vi "get_TIFF_Page.vi"(8 "error in (no error)":errorcluster, 10 "page":i32, 11 "path in":path) -> (0 "error out":errorcluster, 1 "data 32bit":u32[][](array[numeric]), 2 "data 16bit":u16[][](array[numeric]), 3 "path out":path, 4 "bits per sample":u16, 5 "data 8bit":u8[][](array[numeric]), 6 "samples per pixel":i32)   [LabVIEW 2010, in "TIFFManagement.lvlib"]
uses:
  TIFFManagement.lvlib
  VisualCPP/Release/TIFFManagement.dll
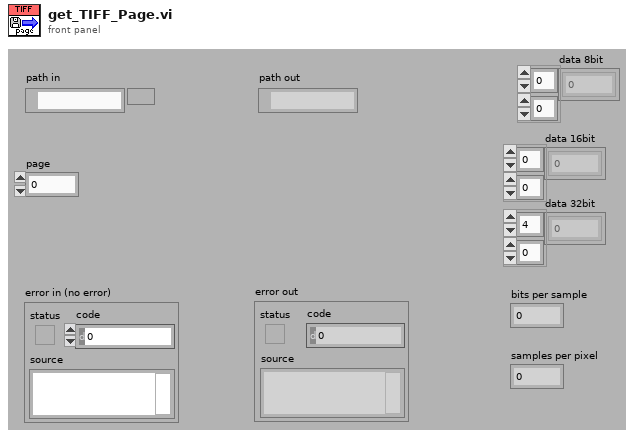
[diagram p1: front panel]
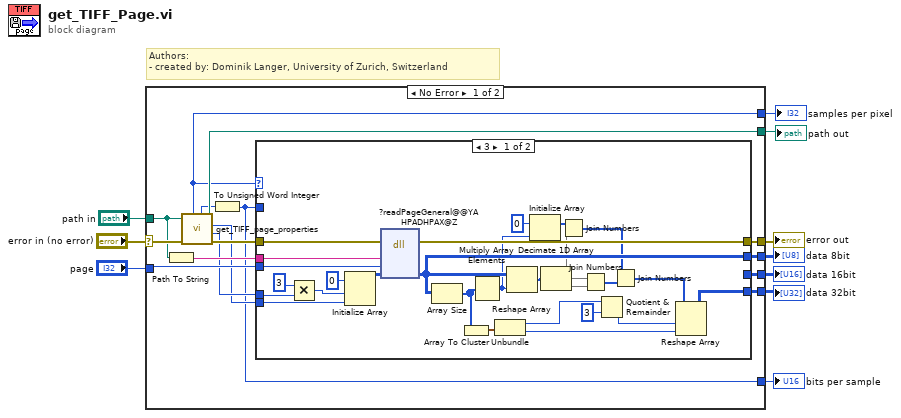
[diagram p0: block diagram]
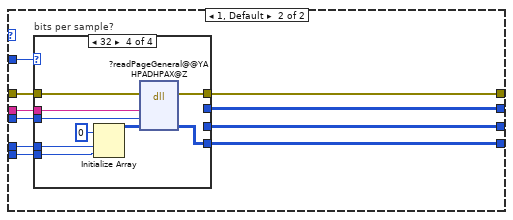
[diagram p2: hidden frame]
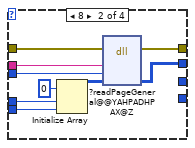
[diagram p4: hidden frame]
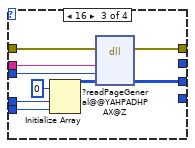
[diagram p5: hidden frame]
diagram:
  # "Authors: \n- created by: Dominik Langer, University of Zurich, Switzerland"
  n1 = case shown="No Error" "error in (no error)" {
    selector: "error in (no error)" -> [w23 w93]
    tunnel: "path in" -> [w21 w92]
    tunnel: "page" -> [w19 _]
    tunnel: [w25 w93] -> w7
    tunnel: [w20 w92] -> w6
    tunnel: [w16 _] -> w5
    tunnel: [w15 _] -> w4
    tunnel: [w14 _] -> w3
    tunnel: [w12 _] -> w2
    tunnel: [w11 _] -> w1
    frame No Error {
      n2 = Path To String(path=w21) -> (string=w24:string)
      n3 = call "get_TIFF_page_properties.vi"("error in (no error)"=w23, "path in"=w21) -> ("error out"=w22:errorcluster, "height"=w18:i32, "width"=w17:i32, "path out"=w20:path, "bits per sample"=w13:i32, "samples per pixel"=w11:i32)  [unwired: 3 in, 1 out]
      n4 = To Unsigned Word Integer(number=w13) -> (unsigned 16bit integer=w12:u16)
      n5 = case shown="3" w11 {
        tunnel: [w52 w63] -> w25
        tunnel: w24 -> [w50 w62]
        tunnel: w22 -> [w53 w61]
        tunnel: w19 -> [w49 w60]
        tunnel: w18 -> [w46 w59]
        tunnel: w17 -> [w51 w58]
        tunnel: [_ w57] -> w16
        tunnel: [w39 w56] -> w15
        tunnel: [w37 w55] -> w14
        tunnel: w12 -> [_ w54]
        frame 3 {
          n6 = Multiply(x=3 ("y"), y=w46) -> (x*y=w45:i32)
          n7 = Initialize Array(u8 0 ("element"), w45, w51) -> (w47:u8[][])
          n8 = dll-call lib="C:/helioscan/common/libraries/TIFFManagement/VisualCPP/Release/TIFFManagement.dll" fn="?readPageGeneral@@YAHPADHPAX@Z"(error in=w53, "path"=w50, "page"=w49, "data"=w47) -> (error out=w52:errorcluster, "data"=w39:u8[][])  [unwired: 5 in, 1 out]
          n9 = Array Size(array=w39) -> (size(s)=w41:i32[])
          n10 = Array To Cluster(array=w41) -> (cluster=w42:cluster{"[0]":i32, "[1]":i32})
          n11 = Multiply Array Elements(1:w41) -> (0:w29:i32)
          n12 = Unbundle(w42) -> ("[0]"=w27:i32, "[1]"=w43:i32)
          n13 = Reshape Array(w39, w29) -> (w40:u8[])
          n14 = Initialize Array(u8 0 ("element"), w29) -> (w31:u8[])
          n15 = Decimate 1D Array(w40) -> (w32:u8[], w36:u8[], w35:u8[])
          n16 = Join Numbers(hi=w31, lo=w32) -> ((hi.lo)=w30:u16[])
          n17 = Join Numbers(hi=w36, lo=w35) -> ((hi.lo)=w34:u16[])
          n18 = Quotient & Remainder(x=w27, y=3) -> (floor(x/y)=w26:i32)  [unwired: 1 out]
          n19 = Join Numbers(hi=w30, lo=w34) -> ((hi.lo)=w38:u32[])
          n20 = Reshape Array(w38, w26, w43) -> (w37:u32[][])
        }
        frame 1, Default {
          n21 = case "bits per sample?" shown="32" w54 {
            tunnel: [w64 w71 w82 w91] -> w63
            tunnel: w62 -> [_ w69 w81 w86]
            tunnel: w61 -> [w64 w70 w80 w90]
            tunnel: w60 -> [_ w68 w79 w87]
            tunnel: w59 -> [_ w67 w78 w89]
            tunnel: w58 -> [_ w66 w77 w88]
            tunnel: [_ _ w76 _] -> w57
            tunnel: [_ w65 _ _] -> w56
            tunnel: [_ _ _ w85] -> w55
            frame Default {
            }
            frame 8 {
              n22 = Initialize Array(u8 0 ("element"), w67, w66) -> (w72:u8[][])
              n23 = dll-call lib="C:/helioscan/common/libraries/TIFFManagement/VisualCPP/Release/TIFFManagement.dll" fn="?readPageGeneral@@YAHPADHPAX@Z"(error in=w70, "path"=w69, "page"=w68, "data"=w72) -> (error out=w71:errorcluster, "data"=w65:u8[][])  [unwired: 5 in, 1 out]
            }
            frame 16 {
              n24 = Initialize Array(u16 0 ("element"), w78, w77) -> (w74:u16[][])
              n25 = dll-call lib="C:/helioscan/common/libraries/TIFFManagement/VisualCPP/Release/TIFFManagement.dll" fn="?readPageGeneral@@YAHPADHPAX@Z"(error in=w80, "path"=w81, "page"=w79, "data"=w74) -> (error out=w82:errorcluster, "data"=w76:u16[][])  [unwired: 5 in, 1 out]
            }
            frame 32 {
              n26 = Initialize Array(u32 0 ("element"), w89, w88) -> (w83:u32[][])
              n27 = dll-call lib="C:/helioscan/common/libraries/TIFFManagement/VisualCPP/Release/TIFFManagement.dll" fn="?readPageGeneral@@YAHPADHPAX@Z"(error in=w90, "path"=w86, "page"=w87, "data"=w83) -> (error out=w91:errorcluster, "data"=w85:u32[][])  [unwired: 5 in, 1 out]
            }
          }
        }
      }
    }
    frame Error {
    }
  }
  "error out" <- w7
  "path out" <- w6
  "data 16bit" <- w5
  "data 8bit" <- w4
  "data 32bit" <- w3
  "bits per sample" <- w2
  "samples per pixel" <- w1
